vi "5790A acdc meas.vi"(6 "error in":errorcluster, 8 "progress":T1(ring), 9 "5790A":refnum<visa-resource-name>) -> (0 "error out":errorcluster, 2 "output value":dbl, 3 "Session Out":refnum<visa-resource-name>)   [LabVIEW 2011]
uses:
  <vilib>/Instr/_visa.llb/VISA GPIB Control REN Mode.ctl
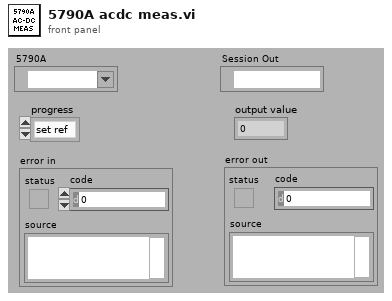
[diagram p1: front panel]
types:
  T1 = enum16{"set ref", "avg ref", "clear ref", "read diff", "read ref"}
  T2 = typedef "VISA GPIB Control REN Mode.ctl" = u16
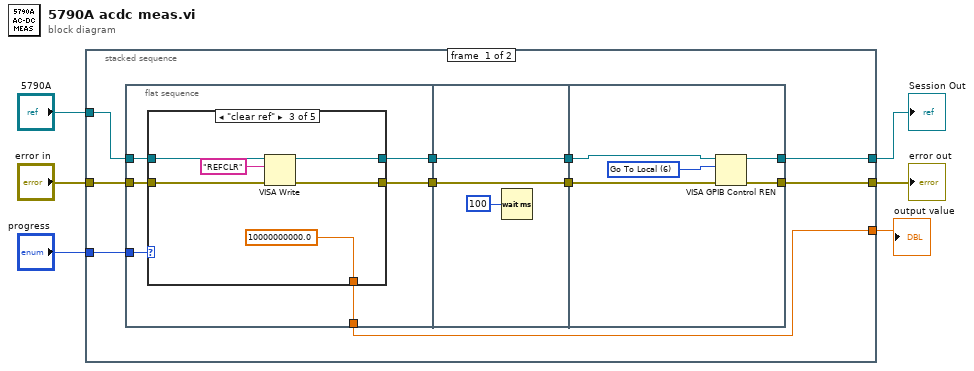
[diagram p0: block diagram]
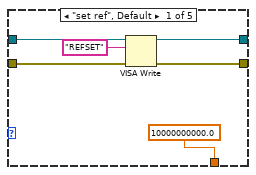
[diagram p2: hidden frame]
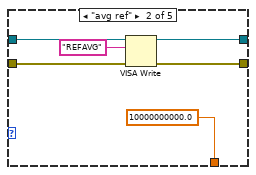
[diagram p3: hidden frame]
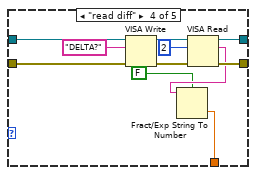
[diagram p4: hidden frame]
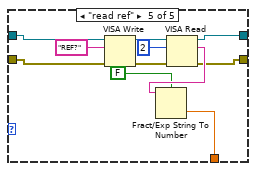
[diagram p5: hidden frame]
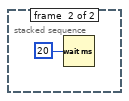
[diagram p6: hidden frame]
diagram:
  n1 = stacked-sequence {
    tunnel: "5790A" -> [w16 _]
    tunnel: "error in" -> [w15 _]
    tunnel: [w14 _] -> w5
    tunnel: [w13 _] -> w6
    tunnel: "progress" -> [w12 _]
    tunnel: [w7 _] -> w1
    frame #0 {
      n2 = flat-sequence {
        tunnel: w12 -> [w22]
        tunnel: w15 -> [w20]
        tunnel: w16 -> [w21]
        tunnel: [w19] -> w10
        tunnel: [w18] -> w8
        tunnel: [w17] -> w7
        tunnel: [w64] -> w11
        tunnel: w10 -> [w64]
        tunnel: [w63] -> w9
        tunnel: w8 -> [w63]
        tunnel: [w69] -> w13
        tunnel: [w68] -> w14
        tunnel: w11 -> [w67]
        tunnel: w9 -> [w66]
        frame #0 {
          n3 = case shown="\"clear ref\"" w22 {
            tunnel: w21 -> [w25 w34 w40 w46 w56]
            tunnel: w20 -> [w26 w33 w39 w47 w55]
            tunnel: [w28 w32 w37 w51 w54] -> w19
            tunnel: [w27 w31 w38 w50 w53] -> w18
            tunnel: [10000000000.0 10000000000.0 10000000000.0 w41 w52] -> w17
            frame "set ref", Default {
              n4 = VISA Write(VISA resource name=w25, write buffer="REFSET", error in (no error)=w26) -> (VISA resource name out=w28:refnum<visa-resource-name>, error out=w27:errorcluster)  [unwired: 1 out]
            }
            frame "avg ref" {
              n5 = VISA Write(VISA resource name=w34, write buffer="REFAVG", error in (no error)=w33) -> (VISA resource name out=w32:refnum<visa-resource-name>, error out=w31:errorcluster)  [unwired: 1 out]
            }
            frame "clear ref" {
              n6 = VISA Write(VISA resource name=w40, write buffer="REFCLR", error in (no error)=w39) -> (VISA resource name out=w37:refnum<visa-resource-name>, error out=w38:errorcluster)  [unwired: 1 out]
            }
            frame "read diff" {
              n7 = VISA Write(VISA resource name=w46, write buffer="DELTA?", error in (no error)=w47) -> (VISA resource name out=w49:refnum<visa-resource-name>, error out=w48:errorcluster)  [unwired: 1 out]
              n8 = VISA Read(VISA resource name=w49, byte count=u32 2, error in (no error)=w48) -> (VISA resource name out=w51:refnum<visa-resource-name>, read buffer=w43:string, error out=w50:errorcluster)  [unwired: 1 out]
              n9 = Fract/Exp String To Number(use system decimal point (T)=FALSE, string=w43) -> (number=w41:dbl)  [unwired: 2 in, 1 out]
            }
            frame "read ref" {
              n10 = VISA Write(VISA resource name=w56, write buffer="REF?", error in (no error)=w55) -> (VISA resource name out=w62:refnum<visa-resource-name>, error out=w61:errorcluster)  [unwired: 1 out]
              n11 = VISA Read(VISA resource name=w62, byte count=u32 2, error in (no error)=w61) -> (VISA resource name out=w54:refnum<visa-resource-name>, read buffer=w58:string, error out=w53:errorcluster)  [unwired: 1 out]
              n12 = Fract/Exp String To Number(use system decimal point (T)=FALSE, string=w58) -> (number=w52:dbl)  [unwired: 2 in, 1 out]
            }
          }
        }
        frame #1 {
          n13 = Wait (ms)(milliseconds to wait=u32 100 ("millisecond multiple")) -> ()  [unwired: 1 out]
        }
        frame #2 {
          w70 = T2 6 items=["Deassert REN", "Assert REN", "Go To Local; Deassert REN ", "Assert REN; Address Device", "Local Lockout (Addressed Devices)", "Local Lockout (This Device)", "Go To Local"] ("Mode")
          n14 = VISA GPIB Control REN(8:w66, 10:w70, 11:w67) -> (0:w68:errorcluster, 3:w69:refnum<visa-resource-name>)
        }
      }
    }
    frame #1 {
      n15 = Wait (ms)(milliseconds to wait=u32 20 ("millisecond multiple")) -> ()  [unwired: 1 out]
    }
  }
  "Session Out" <- w6
  "error out" <- w5
  "output value" <- w1
